vi "PicoScope6000aRunBlock.vi"(7 "Acquisition Settings":T1={"preTriggerSamples"=0, "postTriggerSamples"=1000, "timebase"=2} {"postTriggerSamples" format="%_6p"; "preTriggerSamples" format="%_6p"}, 8 "error in (no error)":errorcluster, 11 "handle in":i16) -> (0 "error out":errorcluster, 3 "handle out":i16, 4 "timeIndisposedMs":dbl, 6 "Total Requested Samples":u64)   [LabVIEW 2010]
doc: "Calls ps6000aRunBlock"
uses:
  ps6000a.dll
  shared/Acquisition Settings.ctl
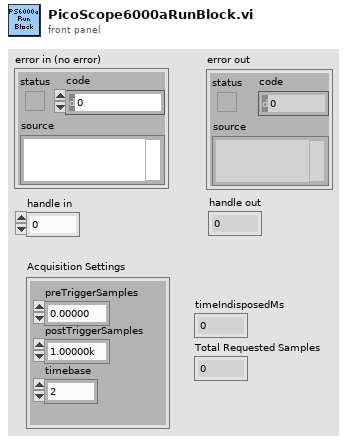
[diagram p1: front panel]
types:
  T1 = typedef "Acquisition Settings.ctl" = cluster{"preTriggerSamples":u64, "postTriggerSamples":u64, "timebase":u32}
  T2 = cluster{"status":bool, "code":u32, "source":string}
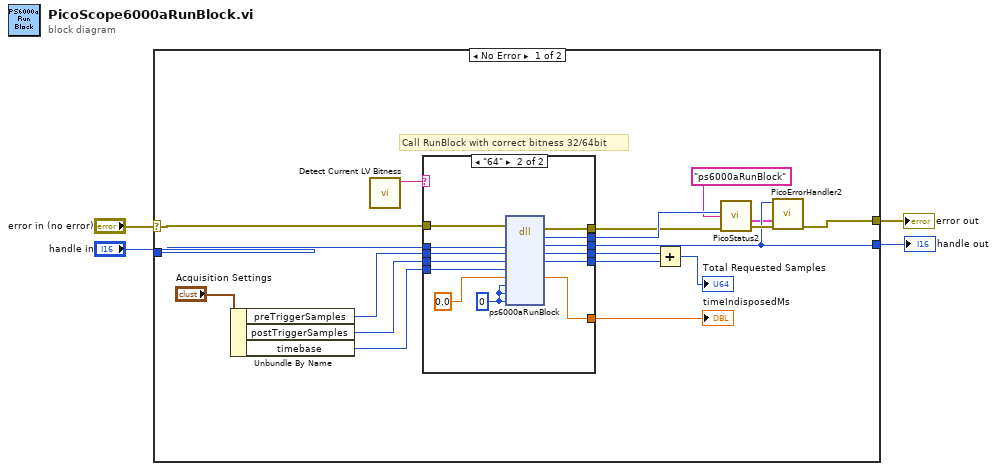
[diagram p0: block diagram]
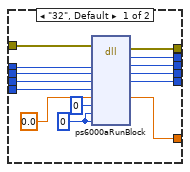
[diagram p2: hidden frame]
diagram:
  n1 = case shown="No Error" "error in (no error)" {
    selector: "error in (no error)" -> [w16 w51]
    tunnel: [w9 w51] -> w2
    tunnel: "handle in" -> [w15 w50]
    tunnel: [w8 w50] -> w3
    frame No Error {
      # "Call RunBlock with correct bitness 32/64bit"
      n2 = Unbundle By Name("Acquisition Settings") -> ("preTriggerSamples"=w14:u64, "postTriggerSamples"=w13:u64, "timebase"=w12:u32)
      n3 = call "Detect Current LV Bitness.vi"() -> ("bitness"=w10:string)  [unwired: 11 in]
      n4 = case shown="\"64\"" w10 {
        tunnel: [w36 w49] -> w22
        tunnel: [w35 w48] -> w21
        tunnel: [w34 w47] -> w19
        tunnel: [w33 w46] -> w18
        tunnel: w16 -> [w32 w45]
        tunnel: w15 -> [w31 w44]
        tunnel: w14 -> [w29 w42]
        tunnel: w13 -> [w28 w41]
        tunnel: w12 -> [w27 w40]
        tunnel: [w26 w39] -> w8
        tunnel: [w23 w37] -> w7
        frame "32", Default {
          w25 = u32 0 ("pParameter")
          n5 = dll-call lib="ps6000a.dll" fn="ps6000aRunBlock" ("ps3000.dll:_ps3000_open_unit@0")(error in=w32, "handle"=w31, "noOfPreTriggerSamples"=w29, "noOfPostTriggerSamples"=w28, "timebase"=w27, "timeIndisposedMs"=0.0 ("pParameter"), "segmentIndex"=u64 0, "lpReady"=w25, "pParameter"=w25) -> (error out=w33:errorcluster, "PICO_STATUS"=w34:u32, "handle"=w26:i16, "noOfPreTriggerSamples"=w36:u64, "noOfPostTriggerSamples"=w35:u64, "timeIndisposedMs"=w23:dbl)  [unwired: 6 in, 1 out]
        }
        frame "64" {
          w38 = u64 0 ("pParameter")
          n6 = dll-call lib="ps6000a.dll" fn="ps6000aRunBlock" ("ps3000.dll:_ps3000_open_unit@0")(error in=w45, "handle"=w44, "noOfPreTriggerSamples"=w42, "noOfPostTriggerSamples"=w41, "timebase"=w40, "timeIndisposedMs"=0.0 ("pParameter"), "segmentIndex"=w38, "lpReady"=w38, "pParameter"=w38) -> (error out=w46:errorcluster, "PICO_STATUS"=w47:u32, "handle"=w39:i16, "noOfPreTriggerSamples"=w49:u64, "noOfPostTriggerSamples"=w48:u64, "timeIndisposedMs"=w37:dbl)  [unwired: 6 in, 1 out]
        }
      }
      "timeIndisposedMs" <- w7
      n7 = Add(x=w22, y=w21) -> (x+y=→"Total Requested Samples":u64)
      n8 = call "PicoStatus2.vi"("PICO source"="ps6000aRunBlock" ("source"), "Error in"=w18, "PICO STATUS"=w19) -> ("error out"=w11:errorcluster, "PICO_STATUS out"=w5:T2)  [unwired: 5 in]
      n9 = call "PicoErrorHandler2.vi"("error in (no error)"=w11, "PICO_STATUS in"=w5, "handle In"=w8) -> ("error out"=w9:errorcluster)  [unwired: 8 in]
    }
    frame Error {
    }
  }
  "error out" <- w2
  "handle out" <- w3
